vi "host_finalize.vi"(8 "error in":errorcluster) -> (0 "error out":errorcluster)   [LabVIEW 2021]
uses:
  host_global_vars.vi
  <vilib>/Utility/error.llb/Error Cluster From Error Code.vi
  <vilib>/rvi/errors/niLvFpgaAdjustHostInterfaceError.vi
  <vilib>/FPGAPlugInAG/PXIe-7856R/niLvFpga_Close_PXIe-7856R.vi
  <vilib>/rvi/interface/nirviReadWriteControl/nirviReadWriteControl.xnode
  FPGA Bitfiles/openlabspm_FPGATarget_fpgamain_eo-gUZR5D1g.lvbitx
  fpga/fpga_main.vi
  <vilib>/rvi/interface/nirviCloseFPGA/nirviCloseFPGA.xnode
  NiFpgaLv.dll
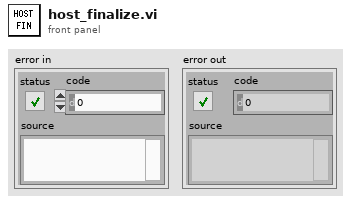
[diagram p1: front panel]
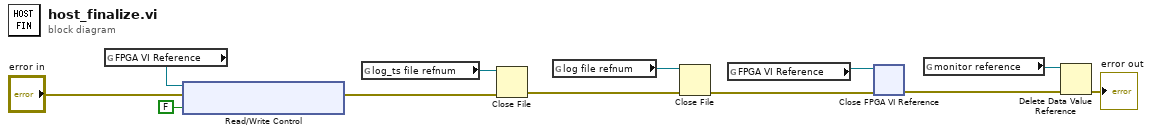
[diagram p0: block diagram]
diagram:
  n1 = global read "host_global_vars.vi" "FPGA VI Reference"() -> (w2:refnum<k20>)
  n2 = xnode "Read/Write Control"("FPGA VI Reference In"=w2, "error in"="error in", "Power"=FALSE ("power")) -> ("error out"=w3:errorcluster)  [unwired: 1 out]
  n3 = global read "host_global_vars.vi" "log_ts file refnum"() -> (w12:refnum<file>)
  n4 = Close File(refnum=w12, error in=w3) -> (error out=w10:errorcluster)  [unwired: 1 out]
  n5 = global read "host_global_vars.vi" "log file refnum"() -> (w11:refnum<file>)
  n6 = Close File(refnum=w11, error in=w10) -> (error out=w8:errorcluster)  [unwired: 1 out]
  n7 = global read "host_global_vars.vi" "FPGA VI Reference"() -> (w9:refnum<k20>)
  n8 = xnode "Close FPGA VI Reference"("FPGA VI Reference In"=w9, "error in"=w8) -> ("error out"=w6:errorcluster)
  n9 = global read "host_global_vars.vi" "monitor reference"() -> (w7:refnum<data-value>)
  n10 = Delete Data Value Reference(data value reference=w7, error in=w6) -> (error out=→"error out":errorcluster)  [unwired: 1 out]
